vi "Acq avvenuta global.vi"() -> ()   [LabVIEW 2019]
panel:
  out "acq auto ammesse?":bool
  out "acq in corso":bool
  out "acq avvenuta":bool
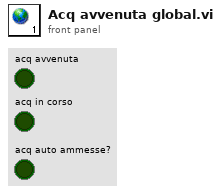
[diagram p1: front panel]
diagram:
